vi "HostEnd.vi"() -> ()   [LabVIEW 2016]
uses:
  <vilib>/Platform/TimedLoop/XDataNode/timing_clust.ctl
  <vilib>/Platform/TimedLoop/XDataNode/nitl_modes.ctl
  <vilib>/Platform/TimedLoop/XDataNode/wakeup.ctl
  <vilib>/express/express analysis/Spectral/Block/exnSpectralBlock spectral measurements power poly.vi
  <vilib>/express/express analysis/Spectral/Block/exnSpectralBlock spectral measurements power WFM.vi
  <vilib>/platform/TimedLoop/XDataNode/XDataNode.xnode
  <vilib>/express/express analysis/Spectral/XNode/ExpressSpectralMeasurementsBlockNode.xnode
  <vilib>/Platform/TimedLoop/XDataNode/XDNodeRunTimeDep.lvlib
panel:
  out "stop or value change":bool
  in  "Fundamental":dbl
  in  "A second":dbl
  in  "Numeric":dbl
  in  "Second Harmonic":dbl
  in  "Third Harmonic":dbl
  in  "Stop":bool
  out "Timed Out":bool
  in  "Upstrum":bool
  in  "Offset b/w notes":dbl
  in  "Working Mode":u16(ring) items=["Brute Force Method", "Guitar Simulation using Karplus-Strong Algorithm"]
  out "Waveform Graph":cluster{"f0":dbl, "df":dbl, "magnitude":dbl[]}(graph)
  in  "volume":dbl(knob)=100.0 scale=4.0..50.0
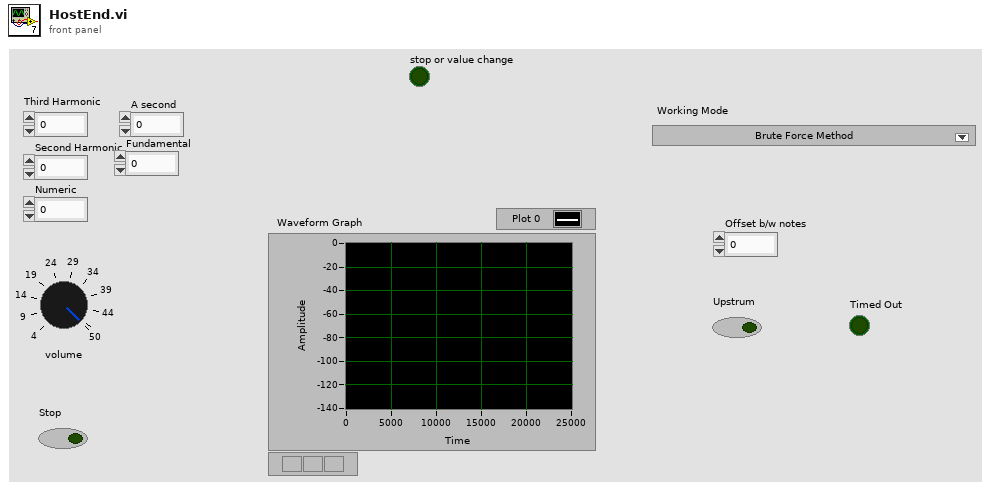
[diagram p1: front panel]
types:
  T1 = cluster{"averaging mode":u16, "weighting mode":u16, "number of averages":u32}
  T2 = cluster{"dB On (F)":bool, "unwrap phase (F)":bool, "convert to degree (F)":bool}
  T3 = typedef "XDNodeRunTimeDep.lvlib/timing_clust.ctl" = cluster{"Expected End [f-1]":u64, "Actual End [f-1]":u64, "Finished Late? [f-1]":bool, "Expected End [i-1]":u64, "Actual End [i-1]":u64, "Finished Late? [i-1]":bool, "Expected Start [i]":u64, "Actual Start [i]":u64, "Expected Start [f]":u64, "Actual Start [f]":u64, "Source Name":string, "Structure Name":string, "Period":i64, "Deadline":i64, "Offset":i64, "Start":i64, "Priority":i32, "Timeout":i32, "Mode":T4, "Wakeup Reason":T5, "Error":errorcluster, "Source Type":string, "Secondary Source Type":string, "Global End Time":u64, "Global Start Time":u64, "Frame Duration":u64, "Iteration Duration":u64, "Assigned CPU":i32, "I/O Scan Engine Mode":u32}
  T4 = typedef "XDNodeRunTimeDep.lvlib/nitl_modes.ctl" = enum32{"No Change", "Process missed periods, maintain original phase", "Discard missed periods, maintain original phase", "Process missed periods, ignore original phase", "Discard missed periods, ignore original phase"}
  T5 = typedef "XDNodeRunTimeDep.lvlib/wakeup.ctl" = enum32{"Normal", "Aborted", "Asynchronous wakeup", "Timing source error", "Timed loop error", "Timeout"}
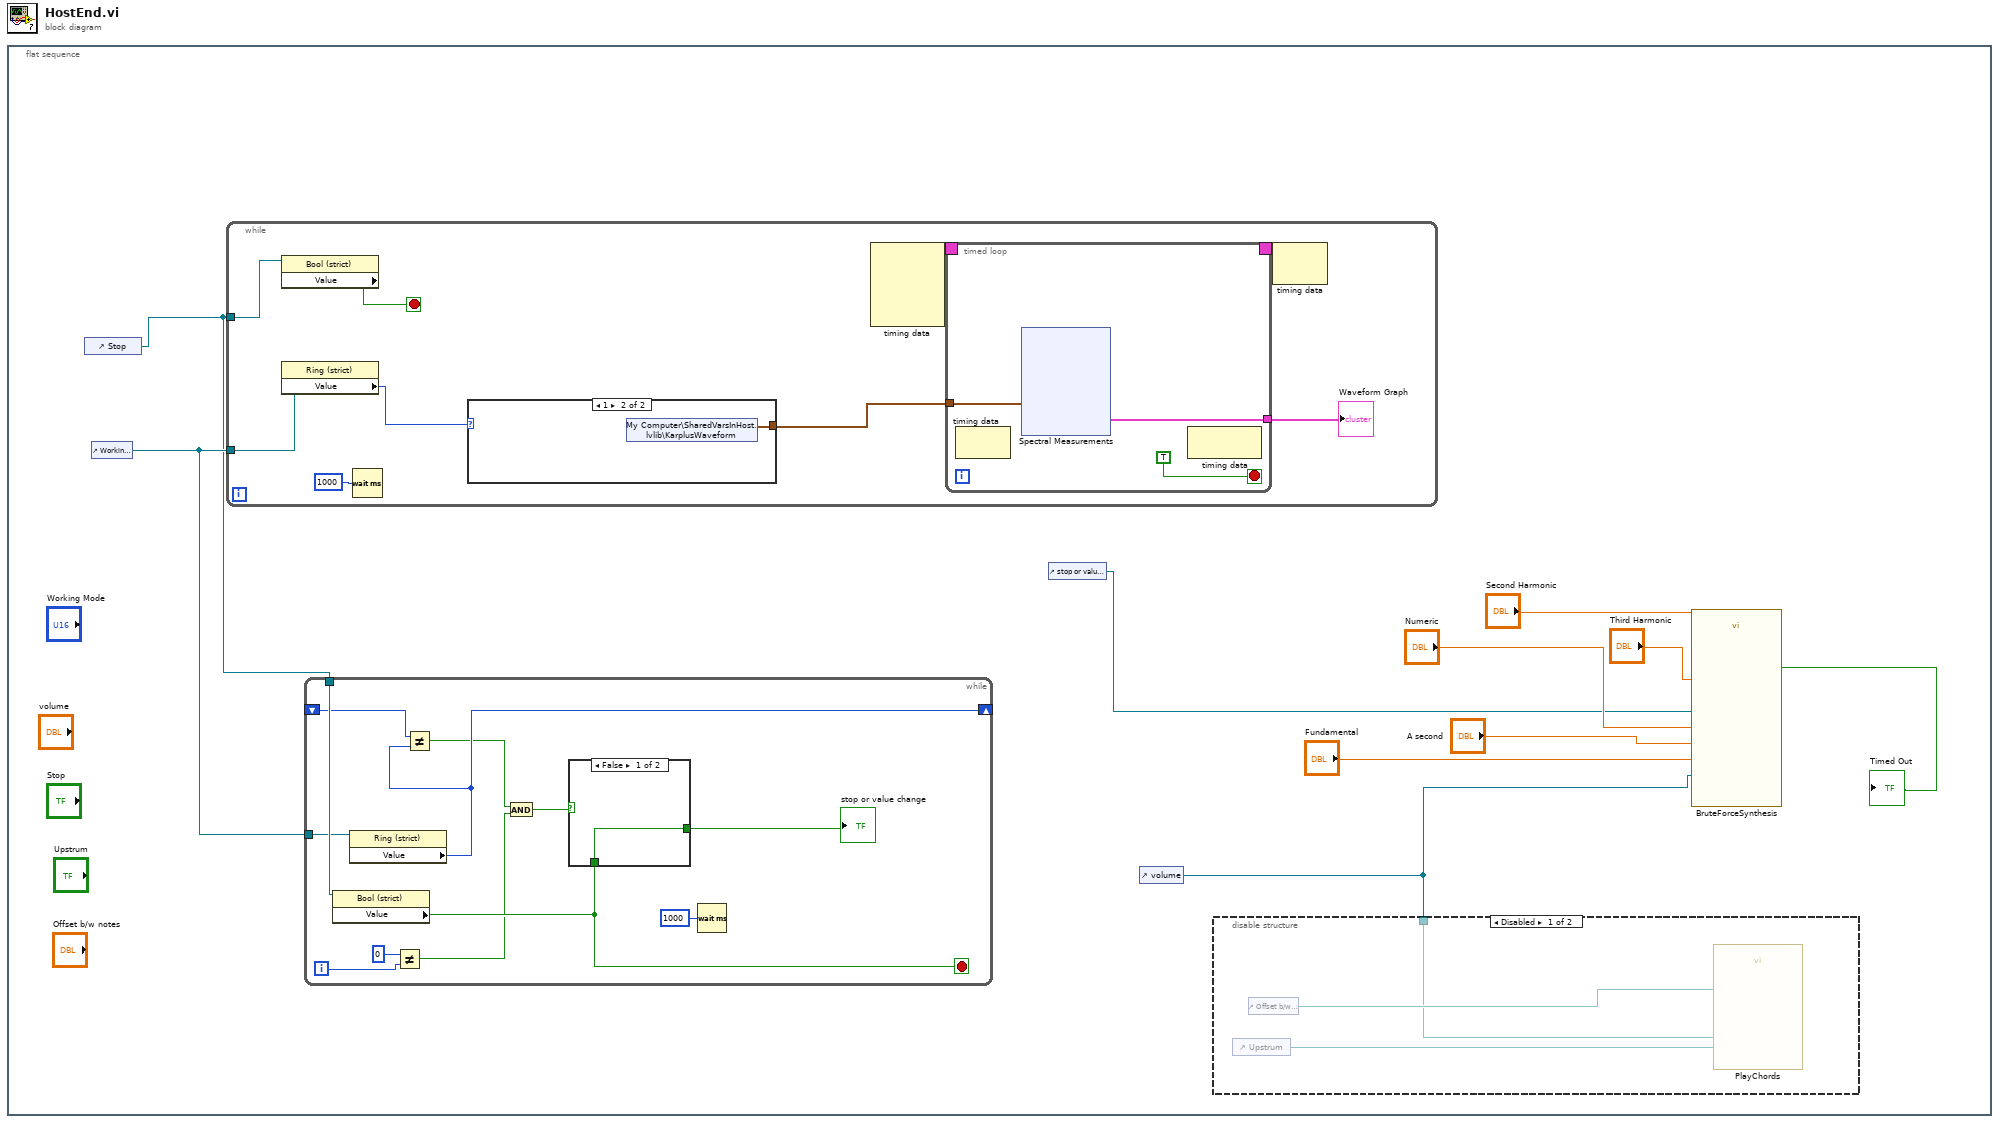
[diagram p0: block diagram]
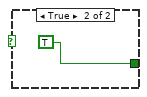
[diagram p3: hidden frame]
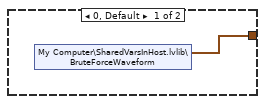
[diagram p4: hidden frame]
diagram:
  n1 = flat-sequence {
    frame #0 {
      n2 = control-ref of="Stop"() -> (w8:refnum<vi>)
      n3 = control-ref of="Working Mode"() -> (w9:refnum<vi>)
      n4 = while {
        tunnel: w8 -> [w31]
        tunnel: w9 -> [w29]
        stop <- w30 stop-if-true
        n5 = property class="Bool (strict)"(reference=w31) -> ("Value"=w30:bool)  [unwired: 1 in, 2 out]
        n6 = property class="Ring (strict)"(reference=w29) -> ("Value"=w28:u16)  [unwired: 1 in, 2 out]
        n7 = Wait (ms)(milliseconds to wait=u32 1000) -> ()  [unwired: 1 out]
        n8 = case shown="1" w28 {
          tunnel: [w37 w38] -> w35
          frame 0, Default {
            n9 = shared-variable "My Computer\\SharedVarsInHost.lvlib\\BruteForceWaveform"() -> (w37:waveform(dbl))  [unwired: 1 in, 1 out]
          }
          frame 1 {
            n10 = shared-variable "My Computer\\SharedVarsInHost.lvlib\\KarplusWaveform"() -> (w38:waveform(dbl))  [unwired: 1 in, 1 out]
          }
        }
        n11 = node-c288() -> (w33:T3)  [unwired: 4 in]
        n12 = timed-loop {
          timing: w33 -> [_]
          timing-out: [_] -> w32
          tunnel: w35 -> [w41]
          tunnel: [w40] -> w34
          stop <- TRUE stop-if-true
          n13 = node-c288() -> ()  [unwired: 1 in, 1 out]
          n14 = xnode "Spectral Measurements"("Signals"=w41) -> ("Power Spectrum"=w40:cluster{"f0":dbl, "df":dbl, "magnitude":dbl[]})  [unwired: 1 in, 1 out]
          n15 = node-c288() -> ()  [unwired: 1 in, 1 out]
        }
        "Waveform Graph" <- w34
        n16 = node-c288(w32) -> ()  [unwired: 1 out]
      }
      n17 = while {
        tunnel: w8 -> [w25]
        shift-right: [w19] -> _
        shift-left: _ -> [w24]
        tunnel: w9 -> [w20]
        i -> [w18]
        stop <- w23 stop-if-true
        n18 = property class="Bool (strict)"(reference=w25) -> ("Value"=w23:bool)  [unwired: 1 in, 2 out]
        n19 = property class="Ring (strict)"(reference=w20) -> ("Value"=w19:u16)  [unwired: 1 in, 2 out]
        n20 = Not Equal?(x=0, y=w18) -> (x != y?=w15:bool)
        n21 = Not Equal?(x=w24, y=w19) -> (x != y?=w16:bool)
        n22 = And(x=w16, y=w15) -> (x .and. y?=w14:bool)
        n23 = case shown="False" w14 {
          tunnel: w23 -> [w26 _]
          tunnel: [w26 TRUE ("x")] -> w22
          frame False {
          }
          frame True {
          }
        }
        "stop or value change" <- w22
        n24 = Wait (ms)(milliseconds to wait=u32 1000) -> ()  [unwired: 1 out]
      }
      n25 = control-ref of="stop or value change"() -> (w1:refnum<vi>)
      n26 = control-ref of="volume"() -> (w2:refnum<vi>)
      n27 = disable-structure shown="Disabled" {
        disable-tunnel: w2 -> [w12 _]
        frame Disabled {
          n28 = control-ref of="Upstrum"() -> (w11:refnum<vi>)
          n29 = control-ref of="Offset b/w notes"() -> (w13:refnum<vi>)
          n30 = call "PlayChords.vi"("Volume"=w12, "Upstrum"=w11, "offset in ms between the string plucking"=w13) -> ()  [unwired: 8 in, 1 out]
        }
        frame Enabled {
        }
      }
      n31 = call "BruteForceSynthesis.vi"("Third Harmonic"="Third Harmonic", "Volume"=w2, "Second Harmonic"="Second Harmonic", "Stop"=w1, "Fundamental"="Fundamental", "A second"="A second", "A third"="Numeric") -> ("timed out?"=→"Timed Out":bool)  [unwired: 3 in, 1 out]
    }
  }
